vi "value2range_VDC.vi"(2 "Voltage [V]":dbl) -> (1 "Limited voltage [V]":dbl, 3 "Negative":bool, 4 "Positive or zero":bool, 5 "Range limit (unsigned) [V]":dbl, 6 "Range limit (signed) [V]":dbl, 7 "Range [-]":i32, 8 "Positive":bool, 9 "Overflow":bool)   [LabVIEW 2020, in "Datron D4xxx.lvlib"]
doc: "This VI gets range from input value for V-DC function. It is used for \"manual autorange\"."
uses:
  Datron D4xxx.lvlib
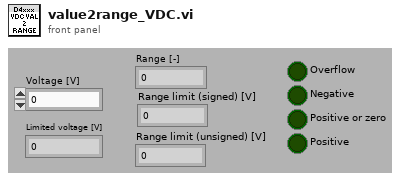
[diagram p1: front panel]
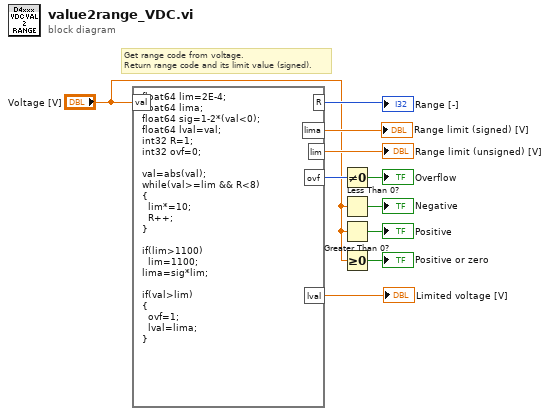
[diagram p0: block diagram]
diagram:
  # "Get range code from voltage.\nReturn range code and its limit value (signed)."
  n1 = formula code="float64 lim=2E-4;\nfloat64 lima;\nfloat64 sig=1-2*(val<0);\nfloat64 lval=val;\nint32 R=1;\nint32 ovf=0;\n\nval=abs(val);\nwhile(val>=lim && R<8)\n{\n  lim*=10;\n  R++;\n}\n\nif(lim>1100)\n  lim=1100;\nlima=sig*lim;\n\nif(val>lim)\n{\n  ovf=1;\n  lval=lima;\n}"("val"="Voltage [V]") -> ("R"=→"Range [-]":i32, "lima"=→"Range limit (signed) [V]":dbl, "lim"=→"Range limit (unsigned) [V]":dbl, "ovf"=w7:i32, "lval"=→"Limited voltage [V]":dbl)
  n2 = Not Equal To 0?(x=w7) -> (x != 0?=→"Overflow":bool)
  n3 = Less Than 0?(x="Voltage [V]") -> (x < 0?=→"Negative":bool)
  n4 = Greater Than 0?(x="Voltage [V]") -> (x > 0?=→"Positive":bool)
  n5 = Greater Or Equal To 0?(x="Voltage [V]") -> (x >= 0?=→"Positive or zero":bool)
